vi "OpenCL Functional Global.vi"(4 "Gain":sgl, 6 "Bias":sgl, 7 "States":T7, 8 "Error In":errorcluster, 10 "Dimension":T1={"Depth"=1, "Height"=1, "Width"=1} {"Width" min=1; "Height" min=1; "Depth" min=1}, 11 "B-Scan":u16[](array[numeric])) -> (0 "Error Out":errorcluster, 1 "Phase":sgl[][][](array[numeric]), 2 "Magnitude":sgl[][][](array[numeric]), 3 "U16 Dimensions":T1={"Depth"=1, "Height"=1, "Width"=1} {"Width" min=1; "Height" min=1; "Depth" min=1})   [LabVIEW 2014]
doc: "A basic starting functional global template for use with OpenCLV. \n\nProvides a functional global with 3 states: Allocate, Operate, and Delete. Also provides a shift register for bundling all OpenCLV memory objects, image objects, and complex function objects.\n\nThis is just a starting point more states can and should be added when appropriate."
uses:
  <vilib>/RaptorView/OpenCLV/Non-User VIs/Allocate Memory/AllocateMemory_u16.vi
  <vilib>/RaptorView/OpenCLV/Non-User VIs/Allocate Memory/AllocateMemory_32f.vi
  <vilib>/RaptorView/OpenCLV/Non-User VIs/FFT/Create FFT Plan 32f.vi
  <vilib>/RaptorView/OpenCLV/Non-User VIs/FFT/FFT Dimension.ctl
  <vilib>/RaptorView/OpenCLV/Non-User VIs/FFT/FFT Types.ctl
  <vilib>/RaptorView/OpenCLV/Non-User VIs/FFT/FFT Direction.ctl
  <vilib>/RaptorView/OpenCLV/Non-User VIs/Set Kernel Arguments/Set Kernel Arguments Memory Object.vi
  <vilib>/RaptorView/OpenCLV/Non-User VIs/Set Kernel Arguments/Set Kernel Arguments 32f.vi
  <vilib>/RaptorView/OpenCLV/Non-User VIs/FFT/Compute FFT 32f.vi
  <vilib>/RaptorView/OpenCLV/Non-User VIs/Read Memory/ReadMemory_32f.vi
  <vilib>/RaptorView/OpenCLV/Non-User VIs/FFT/Delete FFT Plan 32f.vi
  <vilib>/Analysis/NI_AALPro.lvlib
  <vilib>/Analysis/4window.llb/Hanning Window (DBL).vi
  <vilib>/RaptorView/OpenCLV/Non-User VIs/Write Memory/WriteMemory_32f.vi
  <vilib>/RaptorView/OpenCLV/Non-User VIs/Write Memory/WriteMemory_u16.vi
  <vilib>/RaptorView/OpenCLV/Non-User VIs/Controls/Device ID.ctl
  <vilib>/RaptorView/OpenCLV/Non-User VIs/Controls/Memory ID.ctl
  <vilib>/RaptorView/OpenCLV/User Controls/Array Dimensions.ctl
  <vilib>/RaptorView/OpenCLV/Non-User VIs/Controls/Memory Type.ctl
  <vilib>/RaptorView/OpenCLV/Non-User VIs/Controls/Memory Object.ctl
  <vilib>/RaptorView/OpenCLV/Non-User VIs/FFT/FFT Control.ctl
  <vilib>/RaptorView/OpenCLV/Non-User VIs/Controls/Program Handle.ctl
  Memory Typedef.ctl
  OpenCL States.ctl
panel:
  out "x-y 2":u32
  out "x-y":u32
  in  "cluster":T2 {"Phase"."Dimension"."Width" min=1; "Phase"."Dimension"."Height" min=1; "Phase"."Dimension"."Depth" min=1; "Magnitude"."Dimension"."Width" min=1; "Magnitude"."Dimension"."Height" min=1; "Magnitude"."Dimension"."Depth" min=1; "U16 Data"."Dimension"."Width" min=1; "U16 Data"."Dimension"."Height" min=1; "U16 Data"."Dimension"."Depth" min=1; "Pre-FFT Data"."Dimension"."Width" min=1; "Pre-FFT Data"."Dimension"."Height" min=1; "Pre-FFT Data"."Dimension"."Depth" min=1; "Hanning Window Data"."Dimension"."Width" min=1; "Hanning Window Data"."Dimension"."Height" min=1; "Hanning Window Data"."Dimension"."Depth" min=1}
  # "Inputs"
  # "Local OpenCLV Objects"
  # "Outputs"
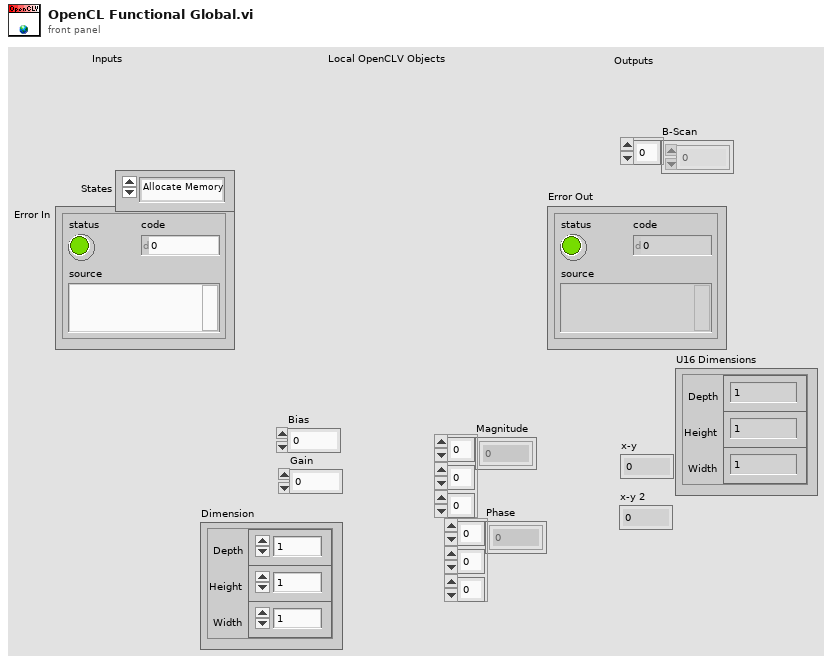
[diagram p1: front panel]
types:
  T1 = typedef "Array Dimensions.ctl" = cluster{"Depth":u64, "Height":u64, "Width":u64}
  T2 = typedef "Memory Typedef.ctl" = cluster{"U16 Data":T3, "Pre-FFT Data":T3, "Hanning Window Data":T3, "Magnitude":T3, "Phase":T3}
  T3 = typedef "OpenCLV x64.lvlib/Memory Object.ctl" = cluster{"Device ID":T4, "Memeroy ID":T5, "Dimension":T1, "Memory Type":T6}
  T4 = typedef "OpenCLV x64.lvlib/Device ID.ctl" = u64
  T5 = typedef "OpenCLV x64.lvlib/Memory ID.ctl" = u64
  T6 = typedef "OpenCLV x64.lvlib/Memory Type.ctl" = enum16{"32f", "u8", "i8", "u16", "i16", "u32", "i32", "64f"}
  T7 = typedef "OpenCL States.ctl" = enum16{"Allocate Memory", "Get U16 Memory Dimension", "Compile Kernels", "Create Device", "Write", "Read", "Operate", "Delete Memory", "Delete"}
  T8 = typedef "OpenCLV x64.lvlib/FFT Direction.ctl" = enum16{"Forward", "Reverse"}
  T9 = typedef "OpenCLV x64.lvlib/FFT Types.ctl" = enum16{"Real to Hermitian", "Hermitian to Real", "Complex to Complex"}
  T10 = typedef "OpenCLV x64.lvlib/FFT Dimension.ctl" = enum16{"1D FFT", "2D FFT", "3D FFT"}
  T11 = typedef "OpenCLV x64.lvlib/Program Handle.ctl" = u64
  T12 = typedef "OpenCLV x64.lvlib/FFT Control.ctl" = cluster{"Device ID":T4, "FFT Types":T9, "FFT Dim":T10, "Real":T3, "Imag":T3, "FFT Plan":u64, "FFT Direction":T8}
  T13 = typedef "OpenCLV x64.lvlib/Kernel Handle.ctl" = u64
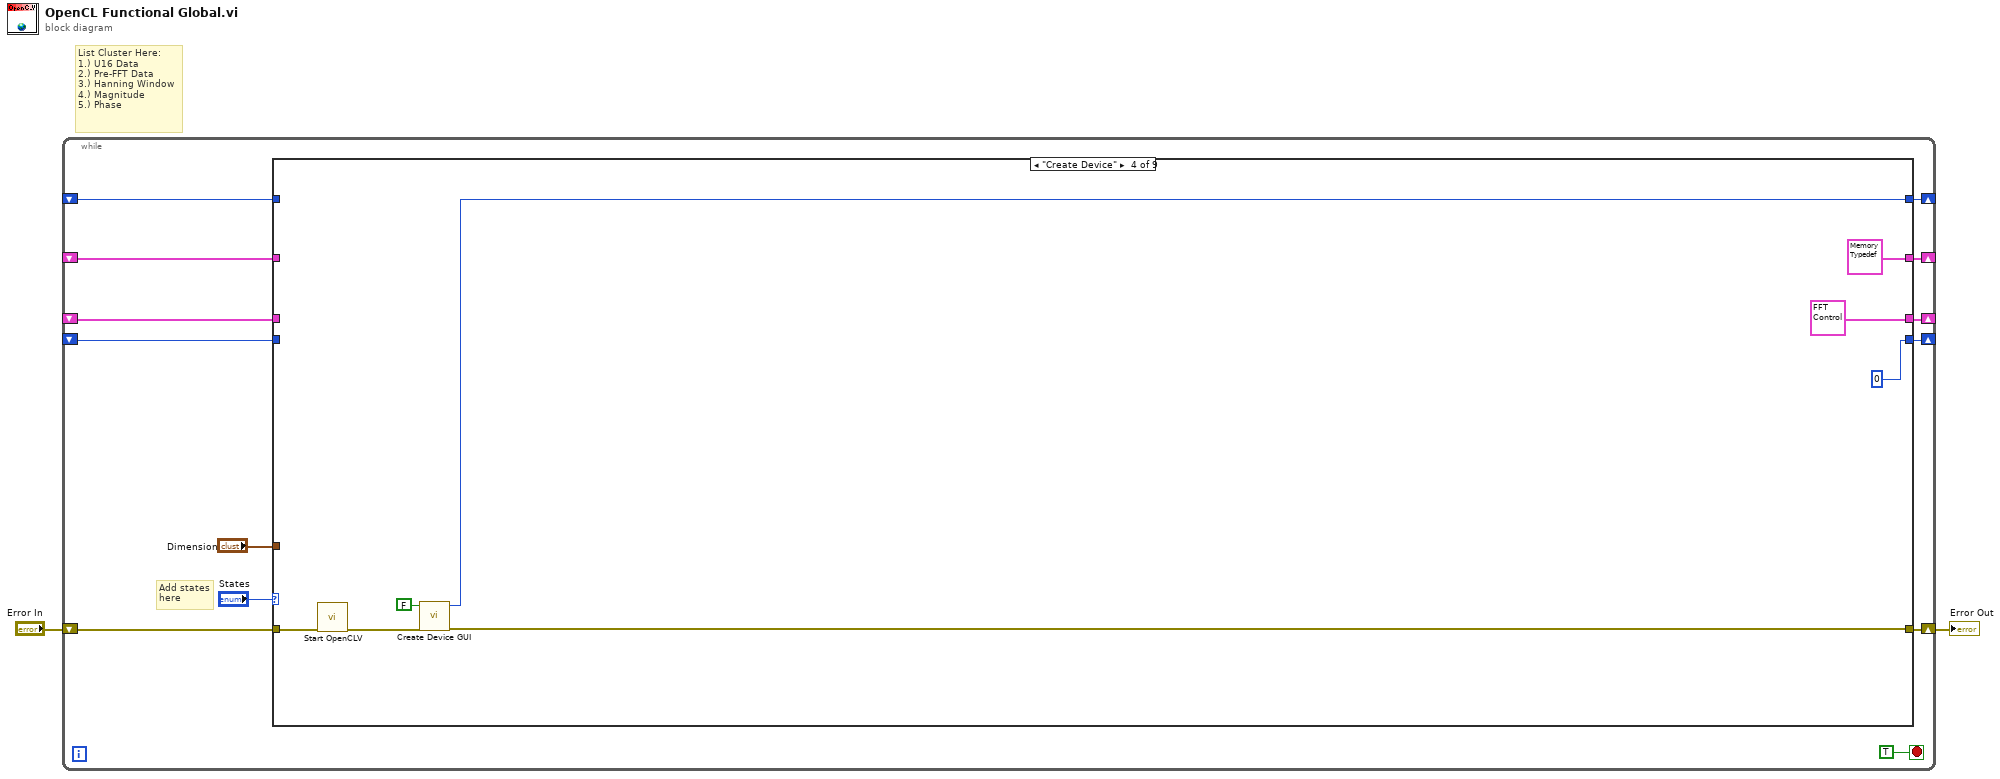
[diagram p0: block diagram]
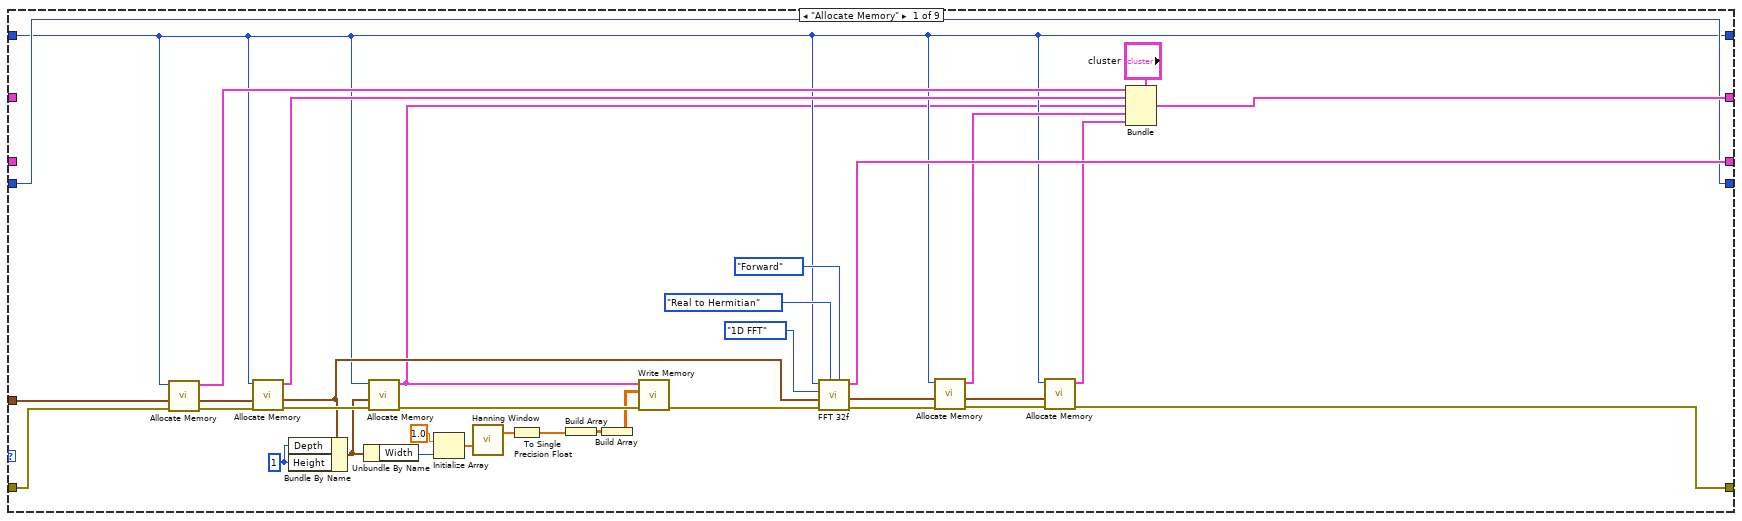
[diagram p2: hidden frame]
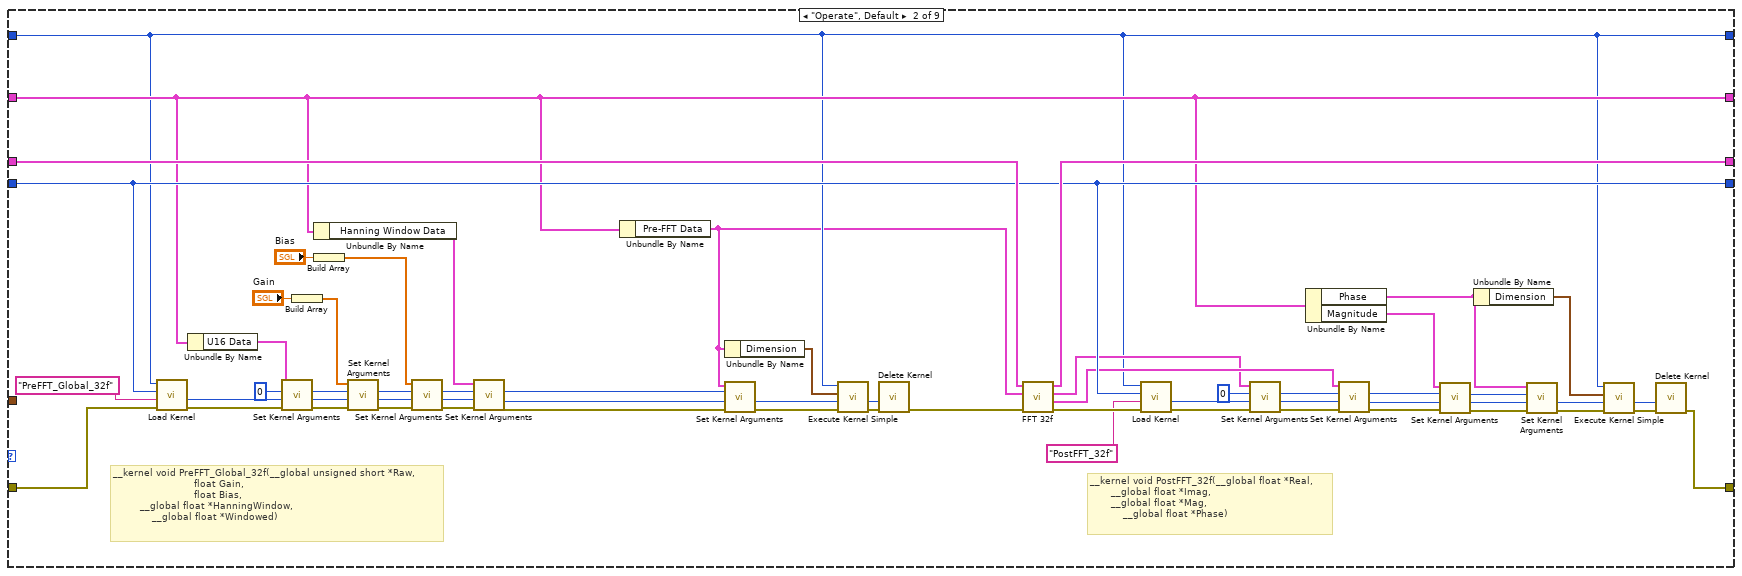
[diagram p3: hidden frame]
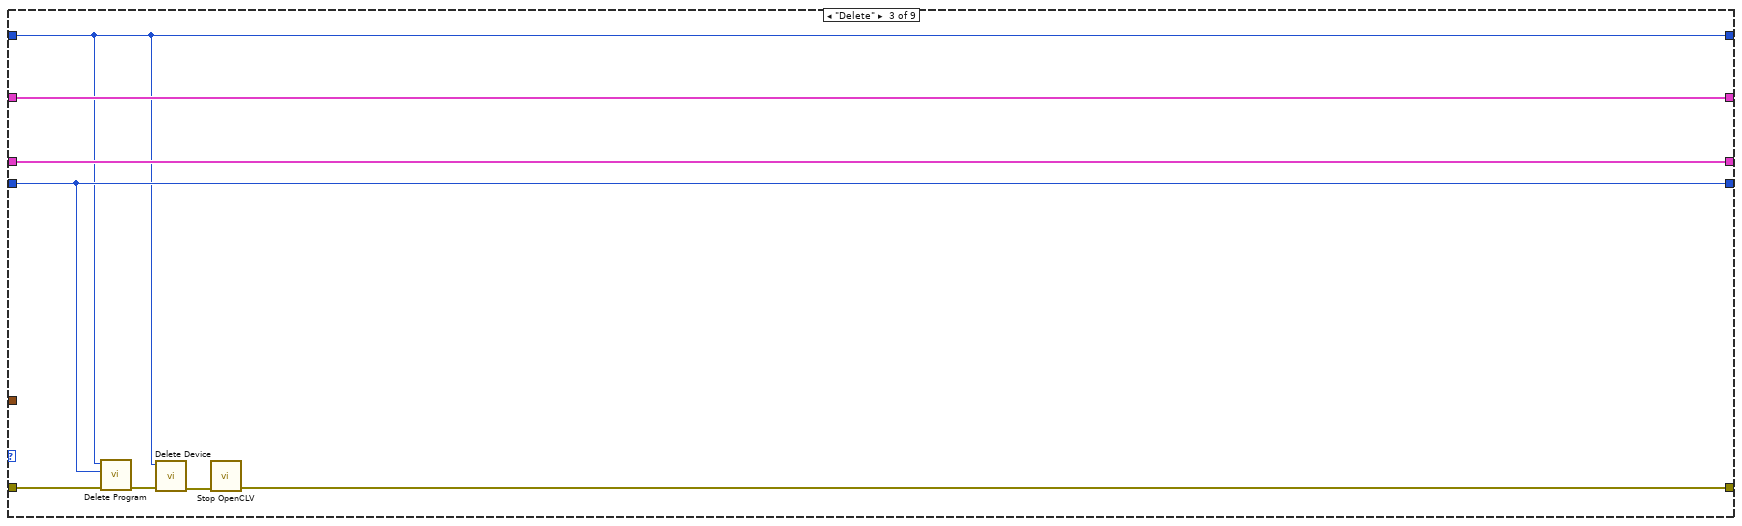
[diagram p4: hidden frame]
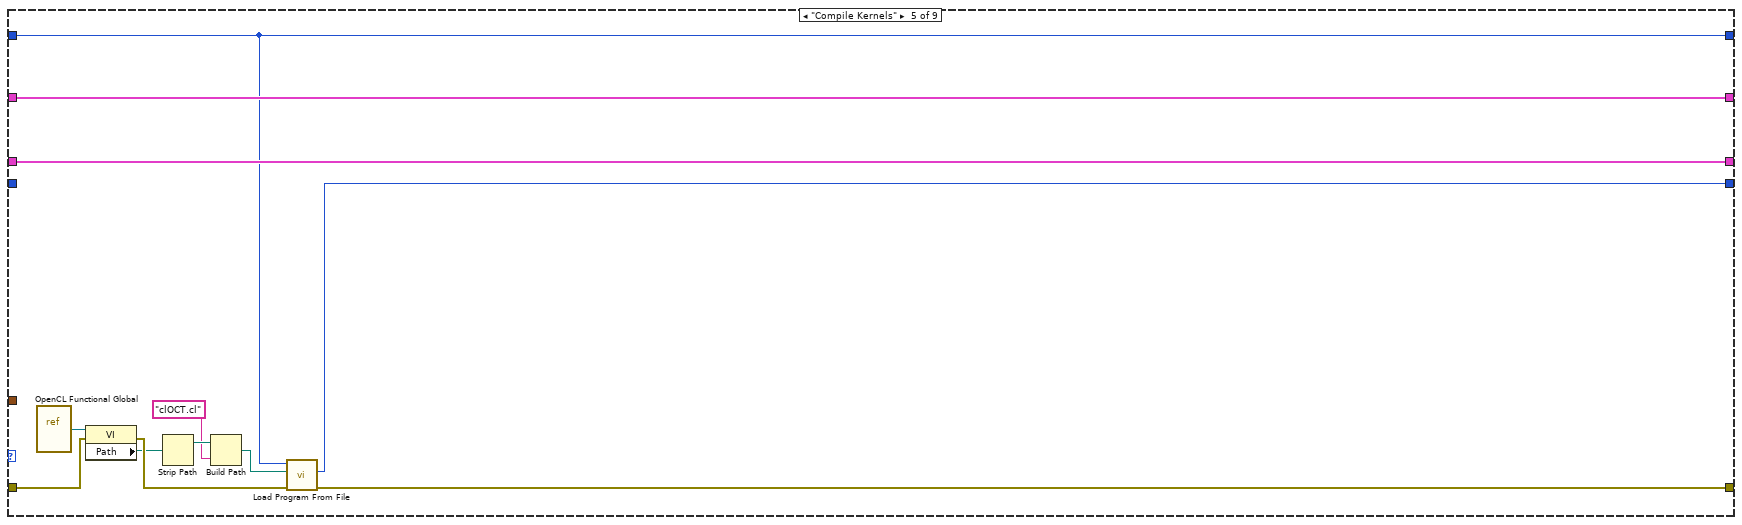
[diagram p5: hidden frame]
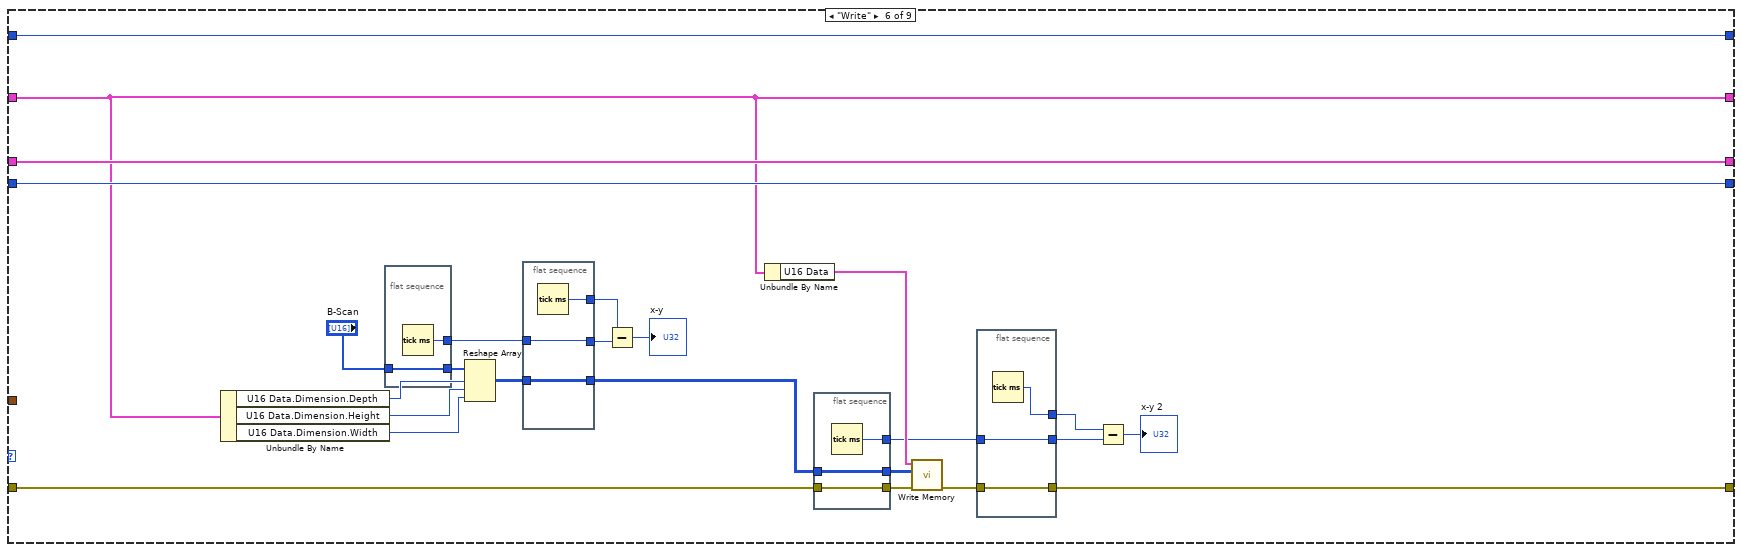
[diagram p6: hidden frame]
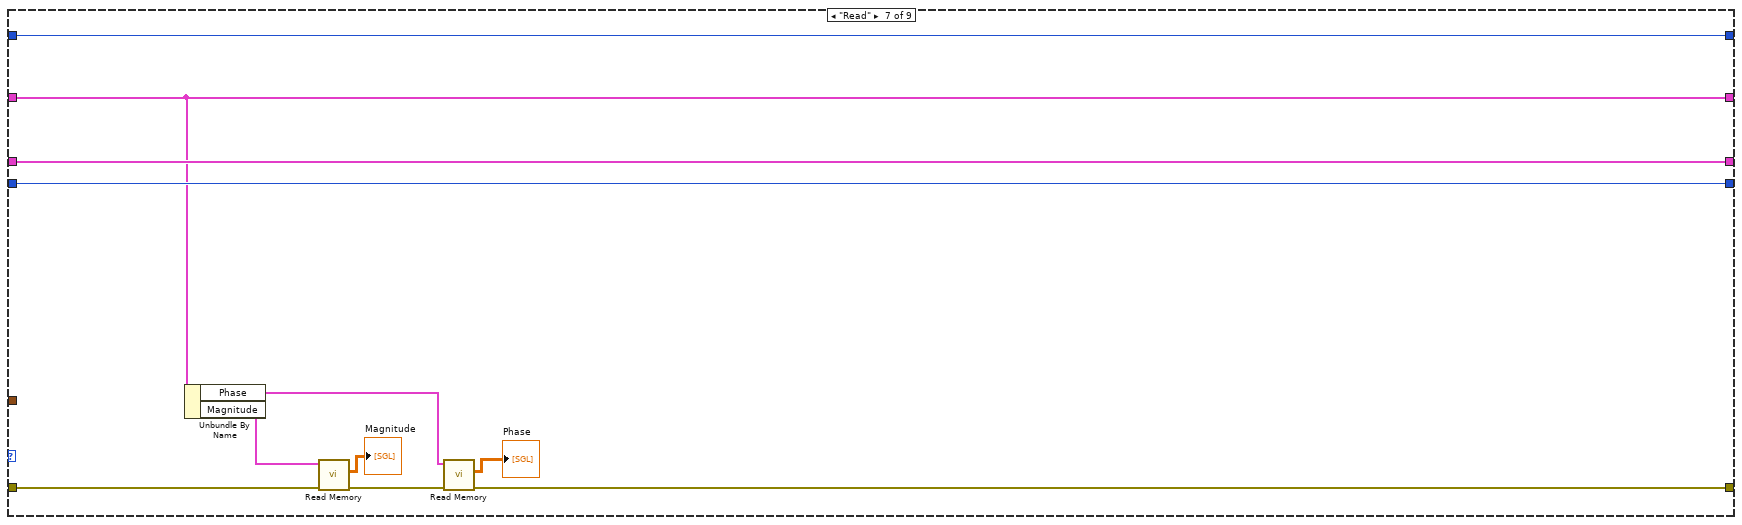
[diagram p7: hidden frame]
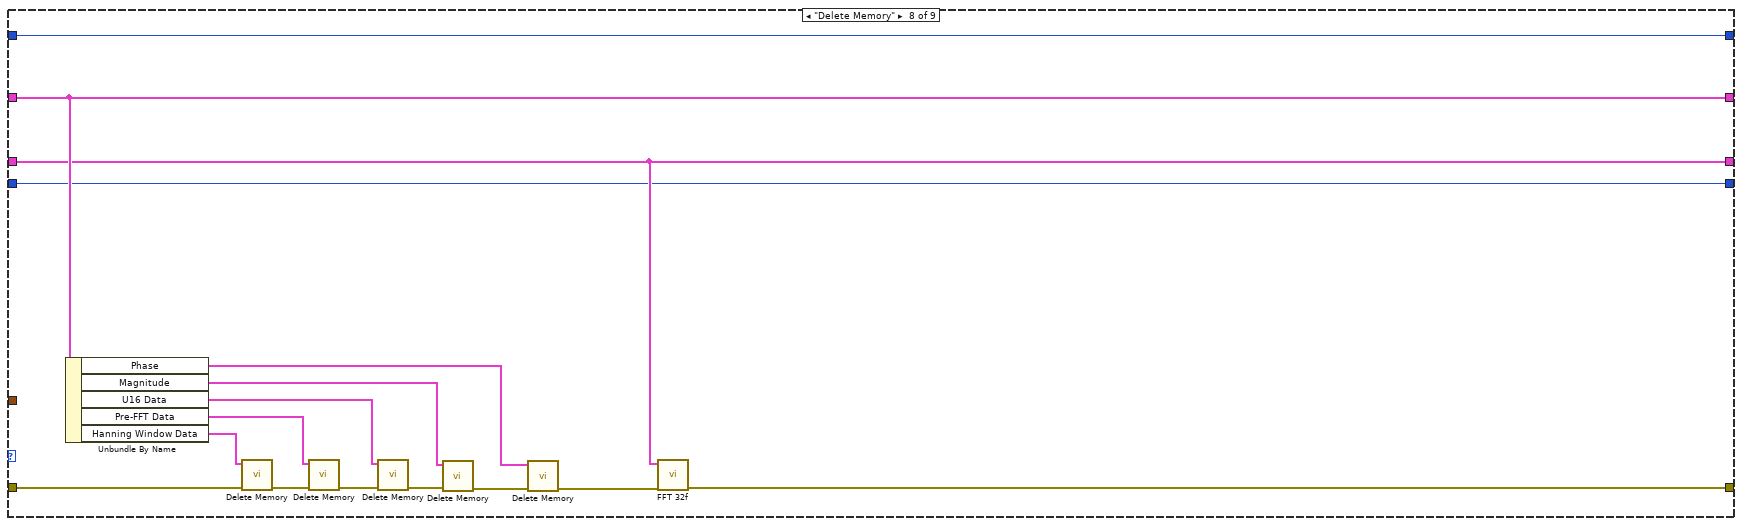
[diagram p8: hidden frame]
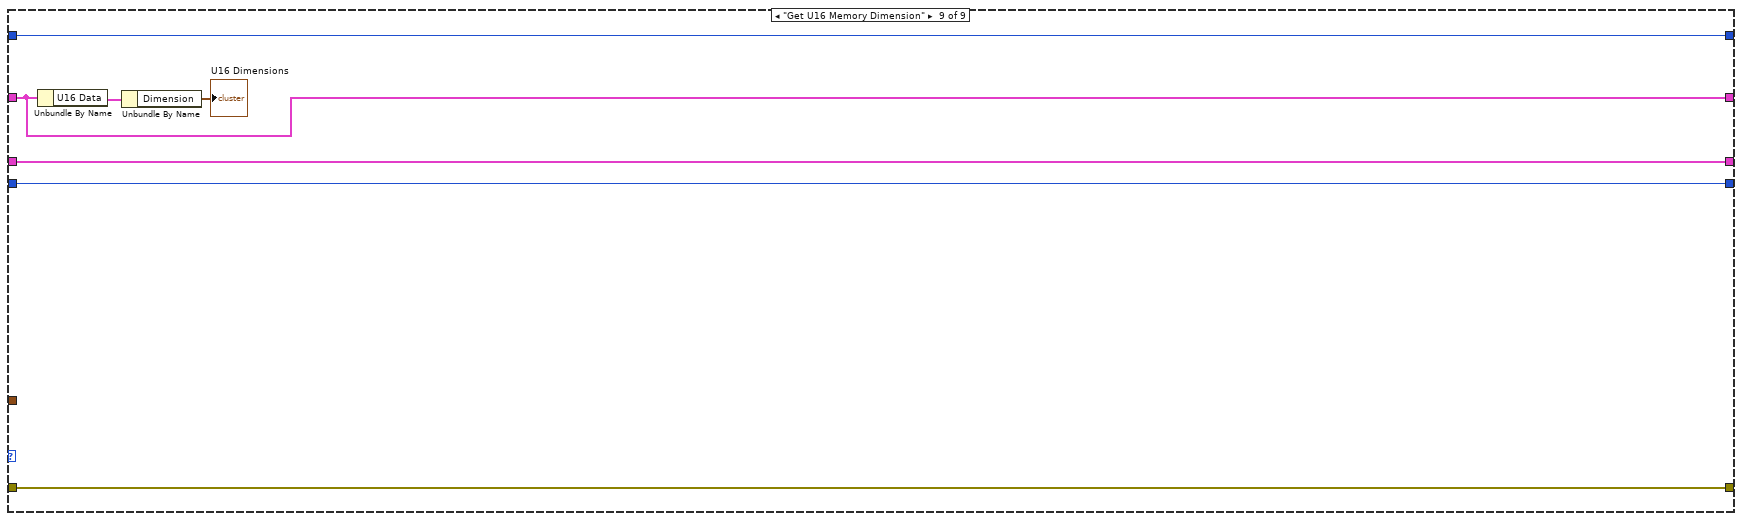
[diagram p9: hidden frame]
diagram:
  # "List Cluster Here:\n1.) U16 Data\n2.) Pre-FFT Data\n3.) Hanning Window\n4.) Magnitude\n5.) Phase"
  n1 = while {
    shift-right: [w14] -> w1
    shift-left: "Error In" -> [w13]
    shift-right: [w10] -> _
    shift-left: _ -> [w11]
    shift-right: [w9] -> _
    shift-left: _ -> [w8]
    shift-right: [w7] -> _
    shift-left: _ -> [w6]
    shift-right: [w5] -> _
    shift-left: _ -> [w4]
    stop <- TRUE stop-if-true
    # "Add states\nhere"
    n2 = case shown="\"Create Device\"" "States" {
      tunnel: [w28 w56 w110 w122 w128 w142 w179 w193 w204] -> w14
      tunnel: w13 -> [w49 w109 w115 w125 w134 w145 w183 w199 w204]
      tunnel: w11 -> [_ w70 w117 _ w137 w158 w176 w192 w201]
      tunnel: [w50 w70 w117 T2 {"U16 Data"={"Device ID"=0, "Memeroy ID"=0, "Dimension"={"Depth"=0, "Height"=0, "Width"=0}, "Memory Type"=enum."32f"}, "Pre-FFT Data"={"Device ID"=0, "Memeroy ID"=0, "Dimension"={"Depth"=0, "Height"=0, "Width"=0}, "Memory Type"=enum."32f"}, "Hanning Window Data"={"Device ID"=0, "Memeroy ID"=0, "Dimension"={"Depth"=0, "Height"=0, "Width"=0}, "Memory Type"=enum."32f"}, "Magnitude"={"Device ID"=0, "Memeroy ID"=0, "Dimension"={"Depth"=0, "Height"=0, "Width"=0}, "Memory Type"=enum."32f"}, "Phase"={"Device ID"=0, "Memeroy ID"=0, "Dimension"={"Depth"=0, "Height"=0, "Width"=0}, "Memory Type"=enum."32f"}} ("cluster") w137 w158 w176 w192 w201] -> w10
      tunnel: [w30 w60 w112 w123 w126 w162 w184 w200 w207] -> w9
      tunnel: w8 -> [w30 w60 w112 _ w126 w162 w184 w200 w207]
      tunnel: [w38 w84 w116 T12 {"Device ID"=0, "FFT Types"=enum."Real to Hermitian", "FFT Dim"=enum."1D FFT", "Real"={"Device ID"=0, "Memeroy ID"=0, "Dimension"={"Depth"=0, "Height"=0, "Width"=0}, "Memory Type"=enum."32f"}, "Imag"={"Device ID"=0, "Memeroy ID"=0, "Dimension"={"Depth"=0, "Height"=0, "Width"=0}, "Memory Type"=enum."32f"}, "FFT Plan"=0, "FFT Direction"=enum."Forward"} ("FFT Object Out") w136 w160 w177 w191 w202] -> w7
      tunnel: w6 -> [_ w85 w116 _ w136 w160 w177 w191 w202]
      tunnel: [w37 w82 w114 T11 0 ("Program Handle") w127 w159 w178 w190 w203] -> w5
      tunnel: w4 -> [w37 w82 w114 _ _ w159 w178 w190 w203]
      tunnel: "Dimension" -> [w16 _ _ _ _ _ _ _ _]
      frame "Allocate Memory" {
        w43 = u64 1 ("Depth")
        n3 = call-poly <vilib>:"Allocate Memory.vi"("Error In"=w49, "Dimension"=w16, "Device In"=w30) -> ("Error Out"=w47:errorcluster, "Dimension Out"=w45:T1, "Memory Object"=w48:T3)  [unwired: 6 in]
        n4 = call-poly <vilib>:"Allocate Memory.vi"("Error In"=w47, "Dimension"=w45, "Device In"=w30) -> ("Error Out"=w44:errorcluster, "Dimension Out"=w42:T1, "Memory Object"=w46:T3)  [unwired: 6 in]
        n5 = Bundle By Name(cluster=w42, "Depth"=w43, "Height"=w43) -> (w25:T1)
        n6 = Unbundle By Name(w25) -> ("Width"=w23:u64)
        n7 = call-poly <vilib>:"Allocate Memory.vi"("Error In"=w44, "Dimension"=w25, "Device In"=w30) -> ("Error Out"=w26:errorcluster, "Memory Object"=w27:T3)  [unwired: 6 in, 1 out]
        n8 = Initialize Array(1.0 ("element"), w23) -> (w24:dbl[])
        n9 = call-poly <vilib>:"Hanning Window.vi"("X"=w24) -> ("Windowed X"=w21:dbl[])  [unwired: 1 out]
        n10 = To Single Precision Float(number=w21) -> (single precision float=w17:sgl[])
        n11 = Build Array(w17) -> (w20:sgl[][])
        n12 = Build Array(w20) -> (w19:sgl[][][])
        n13 = call-poly <vilib>:"Write Memory.vi"("Error In"=w26, "Data In"=w19, "Memory Object In"=w27) -> ("Error Out"=w18:errorcluster)  [unwired: 6 in, 2 out]
        n14 = call-poly <vilib>:"FFT 32f.vi"("Direction"=FFT_Direction."Forward", "FFT Types"=FFT_Types."Real to Hermitian", "Error In"=w18, "Dimension"=w42, "FFT Dimension"=FFT_Dimension."1D FFT", "Labview Device"=w30) -> ("Error Out"=w35:errorcluster, "FFT Output Dimensions"=w34:T1, "FFT Object"=w38:T12)  [unwired: 3 in]
        n15 = call-poly <vilib>:"Allocate Memory.vi"("Error In"=w35, "Dimension"=w34, "Device In"=w30) -> ("Error Out"=w31:errorcluster, "Dimension Out"=w32:T1, "Memory Object"=w33:T3)  [unwired: 6 in]
        n16 = call-poly <vilib>:"Allocate Memory.vi"("Error In"=w31, "Dimension"=w32, "Device In"=w30) -> ("Error Out"=w28:errorcluster, "Memory Object"=w29:T3)  [unwired: 6 in, 1 out]
        n17 = Bundle(cluster="cluster", "U16 Data"=w48, "Pre-FFT Data"=w46, "Hanning Window Data"=w27, "Magnitude"=w33, "Phase"=w29) -> (w50:T2)
      }
      frame "Operate", Default {
        # "__kernel void PostFFT_32f(__global float *Real,\n\t\t\t    __global float *Imag,\n\t\t\t    __global float *Mag,\n    \t\t\t    __global float *Phase)"
        # "__kernel void PreFFT_Global_32f(__global unsigned short *Raw,\n                           float Gain,\n                           float Bias,\n\t\t\t\t\t\t   __global float *HanningWindow,\n\t\t           __global float *Windowed)"
        n18 = call <vilib>:"Load Kernel.vi"("Error In"=w109, "Kernel Name"="PreFFT_Global_32f", "Program Handle"=w82, "Device In"=w60) -> ("Error Out"=w107:errorcluster, "Kernel Handle"=w106:T13)  [unwired: 4 in, 2 out]
        n19 = Unbundle By Name(w70) -> ("U16 Data"=w104:T3)
        n20 = call-poly <vilib>:"Set Kernel Arguments.vi"("Error In"=w107, "Kernel Handle"=w106, "Argument Number"=0, "Memory Object"=w104) -> ("Error Out"=w103:errorcluster, "Kernel Handle out"=w102:T13, "Auto Inc Arugment Number"=w101:i32)  [unwired: 5 in]
        n21 = Build Array("Gain") -> (w100:sgl[])
        n22 = Unbundle By Name(w70) -> ("Hanning Window Data"=w90:T3)
        n23 = Build Array("Bias") -> (w94:sgl[])
        n24 = call-poly <vilib>:"Set Kernel Arguments.vi"("Error In"=w103, "Kernel Handle"=w102, "Argument Number"=w101, "32f Constant"=w100) -> ("Error Out"=w98:errorcluster, "Kernel Handle out"=w97:T13, "Auto Inc Arugment Number"=w96:i32)  [unwired: 5 in]
        n25 = call-poly <vilib>:"Set Kernel Arguments.vi"("Error In"=w98, "Kernel Handle"=w97, "Argument Number"=w96, "32f Constant"=w94) -> ("Error Out"=w93:errorcluster, "Kernel Handle out"=w92:T13, "Auto Inc Arugment Number"=w91:i32)  [unwired: 5 in]
        n26 = call-poly <vilib>:"Set Kernel Arguments.vi"("Error In"=w93, "Kernel Handle"=w92, "Argument Number"=w91, "Memory Object"=w90) -> ("Error Out"=w55:errorcluster, "Kernel Handle out"=w54:T13, "Auto Inc Arugment Number"=w53:i32)  [unwired: 5 in]
        n27 = Unbundle By Name(w70) -> ("Pre-FFT Data"=w52:T3)
        n28 = Unbundle By Name(w52) -> ("Dimension"=w87:T1)
        n29 = call-poly <vilib>:"Set Kernel Arguments.vi"("Error In"=w55, "Kernel Handle"=w54, "Argument Number"=w53, "Memory Object"=w52) -> ("Error Out"=w89:errorcluster, "Kernel Handle out"=w88:T13)  [unwired: 5 in, 1 out]
        n30 = call <vilib>:"Execute Kernel Simple.vi"("Error In"=w89, "Kernel Handle"=w88, "Thread Dimensions"=w87, "Device In"=w60) -> ("Error Out"=w86:errorcluster, "Kernel Handle out"=w59:T13)  [unwired: 4 in, 2 out]
        n31 = call <vilib>:"Delete Kernel.vi"("Error In"=w86, "Kernel In"=w59) -> ("Error Out"=w51:errorcluster)  [unwired: 9 in]
        n32 = call-poly <vilib>:"FFT 32f.vi"("Error In"=w51, "Real In"=w52, "FFT Object"=w85) -> ("Error Out"=w83:errorcluster, "Imag Out"=w74:T3, "Real Out"=w63:T3, "FFT Object Out"=w84:T12)  [unwired: 4 in, 1 out]
        n33 = call <vilib>:"Load Kernel.vi"("Error In"=w83, "Kernel Name"="PostFFT_32f", "Program Handle"=w82, "Device In"=w60) -> ("Error Out"=w80:errorcluster, "Kernel Handle"=w79:T13)  [unwired: 4 in, 2 out]
        n34 = call-poly <vilib>:"Set Kernel Arguments.vi"("Error In"=w80, "Kernel Handle"=w79, "Argument Number"=0, "Memory Object"=w63) -> ("Error Out"=w77:errorcluster, "Kernel Handle out"=w76:T13, "Auto Inc Arugment Number"=w75:i32)  [unwired: 5 in]
        n35 = Unbundle By Name(w70) -> ("Phase"=w62:T3, "Magnitude"=w69:T3)
        n36 = call-poly <vilib>:"Set Kernel Arguments.vi"("Error In"=w77, "Kernel Handle"=w76, "Argument Number"=w75, "Memory Object"=w74) -> ("Error Out"=w73:errorcluster, "Kernel Handle out"=w72:T13, "Auto Inc Arugment Number"=w71:i32)  [unwired: 5 in]
        n37 = call-poly <vilib>:"Set Kernel Arguments.vi"("Error In"=w73, "Kernel Handle"=w72, "Argument Number"=w71, "Memory Object"=w69) -> ("Error Out"=w68:errorcluster, "Kernel Handle out"=w67:T13, "Auto Inc Arugment Number"=w66:i32)  [unwired: 5 in]
        n38 = Unbundle By Name(w62) -> ("Dimension"=w61:T1)
        n39 = call-poly <vilib>:"Set Kernel Arguments.vi"("Error In"=w68, "Kernel Handle"=w67, "Argument Number"=w66, "Memory Object"=w62) -> ("Error Out"=w65:errorcluster, "Kernel Handle out"=w64:T13)  [unwired: 5 in, 1 out]
        n40 = call <vilib>:"Execute Kernel Simple.vi"("Error In"=w65, "Kernel Handle"=w64, "Thread Dimensions"=w61, "Device In"=w60) -> ("Error Out"=w58:errorcluster, "Kernel Handle out"=w57:T13)  [unwired: 4 in, 2 out]
        n41 = call <vilib>:"Delete Kernel.vi"("Error In"=w58, "Kernel In"=w57) -> ("Error Out"=w56:errorcluster)  [unwired: 9 in]
      }
      frame "Delete" {
        n42 = call <vilib>:"Delete Program.vi"("Error In"=w115, "Program In"=w114, "Device ID"=w112) -> ("Error Out"=w113:errorcluster)  [unwired: 8 in]
        n43 = call <vilib>:"Delete Device.vi"("Error In"=w113, "Device In"=w112) -> ("error out"=w111:errorcluster)  [unwired: 9 in]
        n44 = call <vilib>:"Stop OpenCLV.vi"("Error In"=w111) -> ("Error Out"=w110:errorcluster)  [unwired: 10 in]
      }
      frame "Create Device" {
        n45 = call <vilib>:"Start OpenCLV.vi"("Error In"=w125) -> ("Error Out"=w124:errorcluster)  [unwired: 10 in]
        n46 = call <vilib>:"Create Device GUI.vi"("Error In"=w124, "Skip Configuration"=FALSE) -> ("error constant"=w122:errorcluster, "Device Reference"=w123:T4)  [unwired: 8 in]
      }
      frame "Compile Kernels" {
        n47 = vi-ref "OpenCL Functional Global.vi"() -> (w135:refnum<vi>)
        n48 = property class="VI"(reference=w135, error in=w134) -> (error out=w133:errorcluster, "Path"=w132:path)  [unwired: 1 out]
        n49 = Strip Path(path=w132) -> (stripped path=w131:path)  [unwired: 1 out]
        n50 = Build Path(base path=w131, name or relative path="clOCT.cl") -> (appended path=w129:path)
        n51 = call <vilib>:"Load Program From File.vi"("Error In"=w133, "Program Path"=w129, "Device In"=w126) -> ("Error Out"=w128:errorcluster, "Program Handle"=w127:T11)  [unwired: 6 in, 1 out]
      }
      frame "Write" {
        n52 = Unbundle By Name(w158) -> ("U16 Data.Dimension.Depth"=w155:u64, "U16 Data.Dimension.Height"=w156:u64, "U16 Data.Dimension.Width"=w157:u64)
        n53 = flat-sequence {
          tunnel: [w173] -> w154
          tunnel: "B-Scan" -> [w173]
          tunnel: [w172] -> w151
          frame #0 {
            n54 = Tick Count (ms)() -> (millisecond timer value=w172:u32)
          }
        }
        n55 = Reshape Array(w154, w155, w156, w157) -> (w152:u16[][][])
        n56 = flat-sequence {
          tunnel: [w171] -> w146
          tunnel: w152 -> [w171]
          tunnel: [w170] -> w150
          tunnel: w151 -> [w170]
          tunnel: [w169] -> w149
          frame #0 {
            n57 = Tick Count (ms)() -> (millisecond timer value=w169:u32)
          }
        }
        n58 = Subtract(x=w149, y=w150) -> (x-y=→"x-y":u32)
        n59 = Unbundle By Name(w158) -> ("U16 Data"=w161:T3)
        n60 = flat-sequence {
          tunnel: [w165] -> w147
          tunnel: w146 -> [w165]
          tunnel: w145 -> [w164]
          tunnel: [w164] -> w144
          tunnel: [w163] -> w141
          frame #0 {
            n61 = Tick Count (ms)() -> (millisecond timer value=w163:u32)
          }
        }
        n62 = call-poly <vilib>:"Write Memory.vi"("Error In"=w144, "Data In"=w147, "Memory Object In"=w161) -> ("Error Out"=w143:errorcluster)  [unwired: 7 in, 1 out]
        n63 = flat-sequence {
          tunnel: [w168] -> w142
          tunnel: w143 -> [w168]
          tunnel: [w167] -> w140
          tunnel: w141 -> [w167]
          tunnel: [w166] -> w139
          frame #0 {
            n64 = Tick Count (ms)() -> (millisecond timer value=w166:u32)
          }
        }
        n65 = Subtract(x=w139, y=w140) -> (x-y=→"x-y 2":u32)
      }
      frame "Read" {
        n66 = Unbundle By Name(w176) -> ("Phase"=w181:T3, "Magnitude"=w182:T3)
        n67 = call-poly <vilib>:"Read Memory.vi"("Error In"=w183, "Memory Object In"=w182) -> ("Error Out"=w180:errorcluster, "Data Out"=→"Magnitude":sgl[][][])  [unwired: 6 in, 2 out]
        n68 = call-poly <vilib>:"Read Memory.vi"("Error In"=w180, "Memory Object In"=w181) -> ("Error Out"=w179:errorcluster, "Data Out"=→"Phase":sgl[][][])  [unwired: 6 in, 2 out]
      }
      frame "Delete Memory" {
        n69 = Unbundle By Name(w192) -> ("Phase"=w187:T3, "Magnitude"=w188:T3, "U16 Data"=w194:T3, "Pre-FFT Data"=w195:T3, "Hanning Window Data"=w196:T3)
        n70 = call <vilib>:"Delete Memory.vi"("Error In"=w199, "Memory Object In"=w196) -> ("Error Out"=w198:errorcluster)  [unwired: 8 in, 1 out]
        n71 = call <vilib>:"Delete Memory.vi"("Error In"=w198, "Memory Object In"=w195) -> ("Error Out"=w197:errorcluster)  [unwired: 8 in, 1 out]
        n72 = call <vilib>:"Delete Memory.vi"("Error In"=w197, "Memory Object In"=w194) -> ("Error Out"=w189:errorcluster)  [unwired: 8 in, 1 out]
        n73 = call <vilib>:"Delete Memory.vi"("Error In"=w189, "Memory Object In"=w188) -> ("Error Out"=w186:errorcluster)  [unwired: 8 in, 1 out]
        n74 = call <vilib>:"Delete Memory.vi"("Error In"=w186, "Memory Object In"=w187) -> ("Error Out"=w185:errorcluster)  [unwired: 8 in, 1 out]
        n75 = call-poly <vilib>:"FFT 32f.vi"("Error In"=w185, "FFT Object"=w191) -> ("Error Out"=w193:errorcluster)  [unwired: 9 in]
      }
      frame "Get U16 Memory Dimension" {
        n76 = Unbundle By Name(w201) -> ("U16 Data"=w206:T3)
        n77 = Unbundle By Name(w206) -> ("Dimension"=→"U16 Dimensions":T1)
      }
    }
  }
  "Error Out" <- w1
